vi "IDS_system_getFeatureName.vi"(3 "error in (no error)":errorcluster, 4 "featurenumber":i32, 5 "deviceHandle":i32) -> (0 "error out":errorcluster, 1 "featurename out":string, 2 "deviceHandle out":i32)   [LabVIEW 2016]
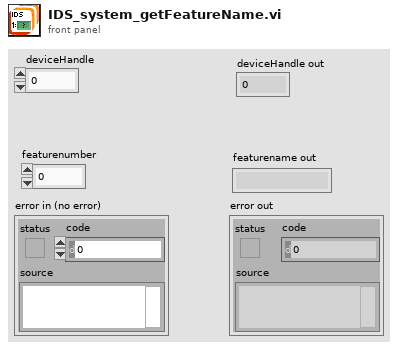
[diagram p1: front panel]
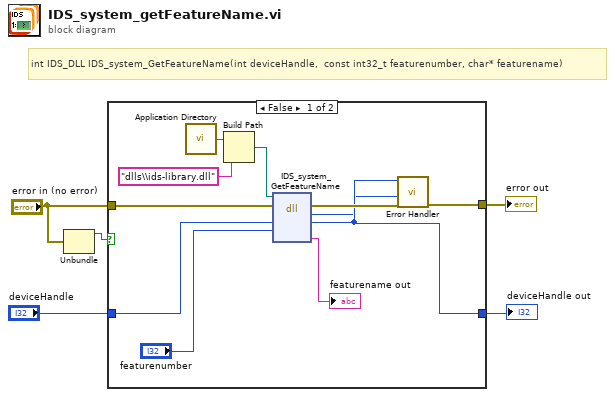
[diagram p0: block diagram]
diagram:
  # "int IDS_DLL IDS_system_GetFeatureName(int deviceHandle,  const int32_t featurenumber, char* featurename)"
  n1 = Unbundle("error in (no error)") -> ("status"=w1:bool)  [unwired: 2 out]
  n2 = case shown="False" w1 {
    tunnel: "error in (no error)" -> [w15 w18]
    tunnel: [w13 w18] -> w5
    tunnel: "deviceHandle" -> [w12 w17]
    tunnel: [w11 w17] -> w3
    frame False {
      n3 = call <vilib>:"Application Directory.vi"() -> ("Application Directory"=w8:path)
      n4 = Build Path(base path=w8, name or relative path="dlls\\ids-library.dll" ("ipAddress")) -> (appended path=w6:path)
      n5 = dll-call lib="C:/Users/matheus/Desktop/LabVIEW_Draft_V1.6.0/dlls/ids-library.*" fn="IDS_system_GetFeatureName"(path in=w6, error in=w15, "deviceHandle"=w12, "featurenumber"="featurenumber") -> (error out=w14:errorcluster, "Rückgabetyp"=w10:i32, "deviceHandle"=w11:i32, "featurename"=→"featurename out":string)  [unwired: 3 in, 1 out]
      n6 = call "Error Handler.vi"("error in (no error)"=w14, "error code"=w10, "deviceHandle"=w11) -> ("error out"=w13:errorcluster)  [unwired: 7 in, 1 out]
    }
    frame True {
    }
  }
  "error out" <- w5
  "deviceHandle out" <- w3
